vi "Add event counter.vi"(8 "error in (no error)":errorcluster caption="entrée d'erreur (pas d'erreur)", 10 "event":refnum<user-event>, 11 "DAQmxTaskContainer en entrée":refnum<class "DAQmxTaskContainer.lvclass">) -> (0 "error out":errorcluster caption="sortie d'erreur", 3 "DAQmxTaskContainer en sortie":refnum<class "DAQmxTaskContainer.lvclass">)   [LabVIEW 2015, in "DAQmxTaskContainer.lvclass"]
uses:
  DAQmxTaskContainer.lvclass
  DAQmxTaskContainer.lvclass/DAQmxTaskContainer.ctl
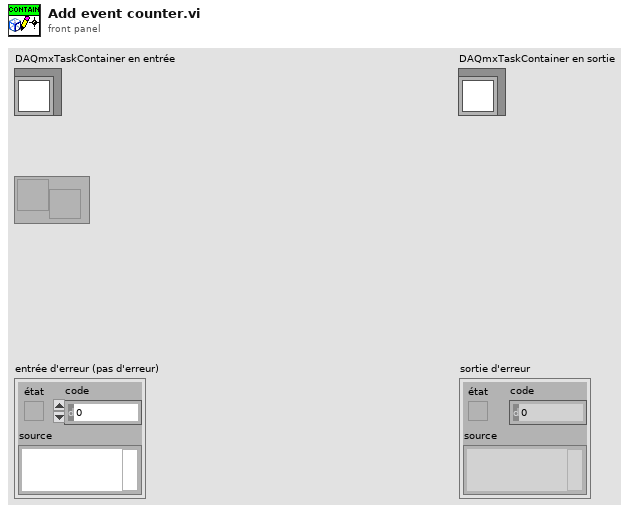
[diagram p1: front panel]
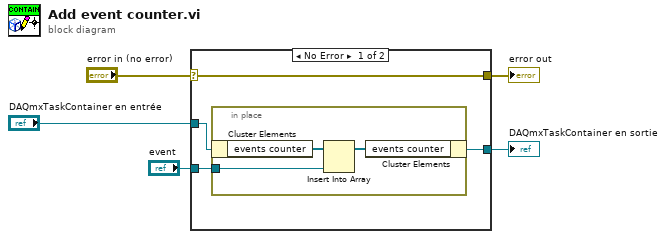
[diagram p0: block diagram]
diagram:
  n1 = case shown="No Error" "error in (no error)" {
    selector: "error in (no error)" -> [w9 w13]
    tunnel: [w9 w13] -> w4
    tunnel: [w6 w14] -> w2
    tunnel: "DAQmxTaskContainer en entrée" -> [w8 w14]
    tunnel: "event" -> [w7 _]
    frame No Error {
      n2 = in-place {
        in-place-border: w7 -> [w11]
        n3 = in-place-cluster #1(w8) -> ("events counter"=w12:refnum<user-event>[])
        n4 = Insert Into Array(array=w12, new element=w11) -> (w10:refnum<user-event>[])  [unwired: 1 in]
        n5 = in-place-cluster #1("events counter"=w10) -> (w6:refnum<class "DAQmxTaskContainer.lvclass">)
      }
    }
    frame Error {
    }
  }
  "error out" <- w4
  "DAQmxTaskContainer en sortie" <- w2
